vi "right2.vi"(10 "Parâmetros Ini 2":T2={"Gyro Port"=0, "Sensor - Left"=3, "Sensor - Right"=2, "     Color \nSensor Port"=1, "Kp Front"=0.5, "Motor speed"=-15, "Distance to street"=0.0, "Motor speed turns"=16, "Kp Curvas"=0.5} {"Kp Front" format="%.3f"; "Color \nSensor Port" items=["Port 1", "Port 2", "Port 3", "Port 4"]; "Sensor - Right" items=["Port 1", "Port 2", "Port 3", "Port 4"]; "Sensor - Left" items=["Port 1", "Port 2", "Port 3", "Port 4"]; "Gyro Port" items=["Port 1", "Port 2", "Port 3", "Port 4"]}, 11 "NXT/EV3":T1) -> (0 "x = y?":bool, 2 "NXT/EV3 2":T1)   [LabVIEW 2016]
uses:
  <vilib>/NXT/Subs/LVHSConnector.ctl
  <vilib>/NXT/LegoClasses/BrickReference/BrickReference.lvclass
  parametros.ctl
  <vilib>/NXT/Block Support/NXT_InputPort.ctl
  <vilib>/NXT/Block Support/NXT_OutputPort.ctl
  <vilib>/NXT/Dual Mode Library/Sensors/EV3_Gyro_Angle.vi
  <vilib>/NXT/NXTIO Xnodes/NXTIONodeSubVIs/NXTMoveMotors.vi
  <vilib>/NXT/NXTIO Xnodes/AddressXNode/NXTIOAddress.xnode
  <vilib>/NXT/NXTIO Xnodes/NXTIOXNode/NXTIO.xnode
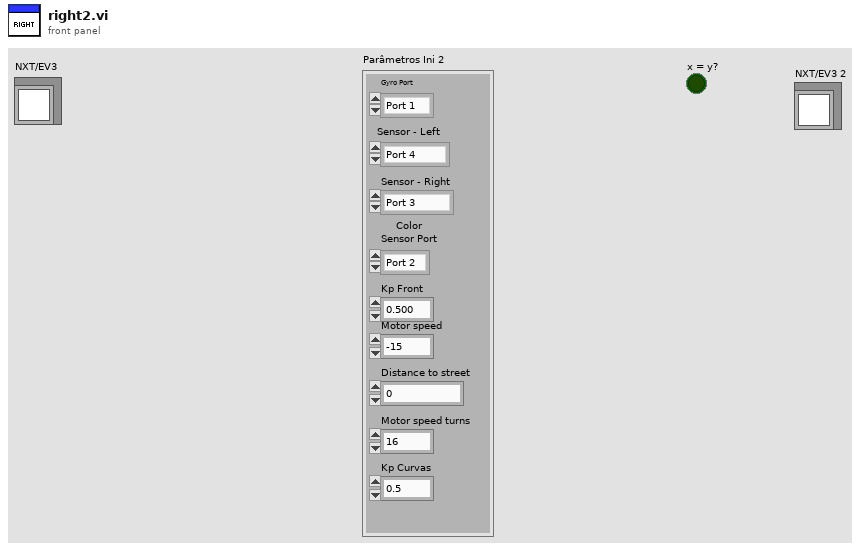
[diagram p1: front panel]
types:
  T1 = typedef "LVHSConnector.ctl" = refnum<class "BrickReference.lvclass">
  T2 = typedef "parametros.ctl" = cluster{"Gyro Port":T3, "Sensor - Left":T3, "Sensor - Right":T3, "     Color \nSensor Port":T3, "Kp Front":dbl, "Motor speed":i32, "Distance to street":dbl, "Motor speed turns":i32, "Kp Curvas":dbl}
  T3 = typedef "NXT_InputPort.ctl" = u32
  T4 = typedef "NXT_OutputPort.ctl" = u8
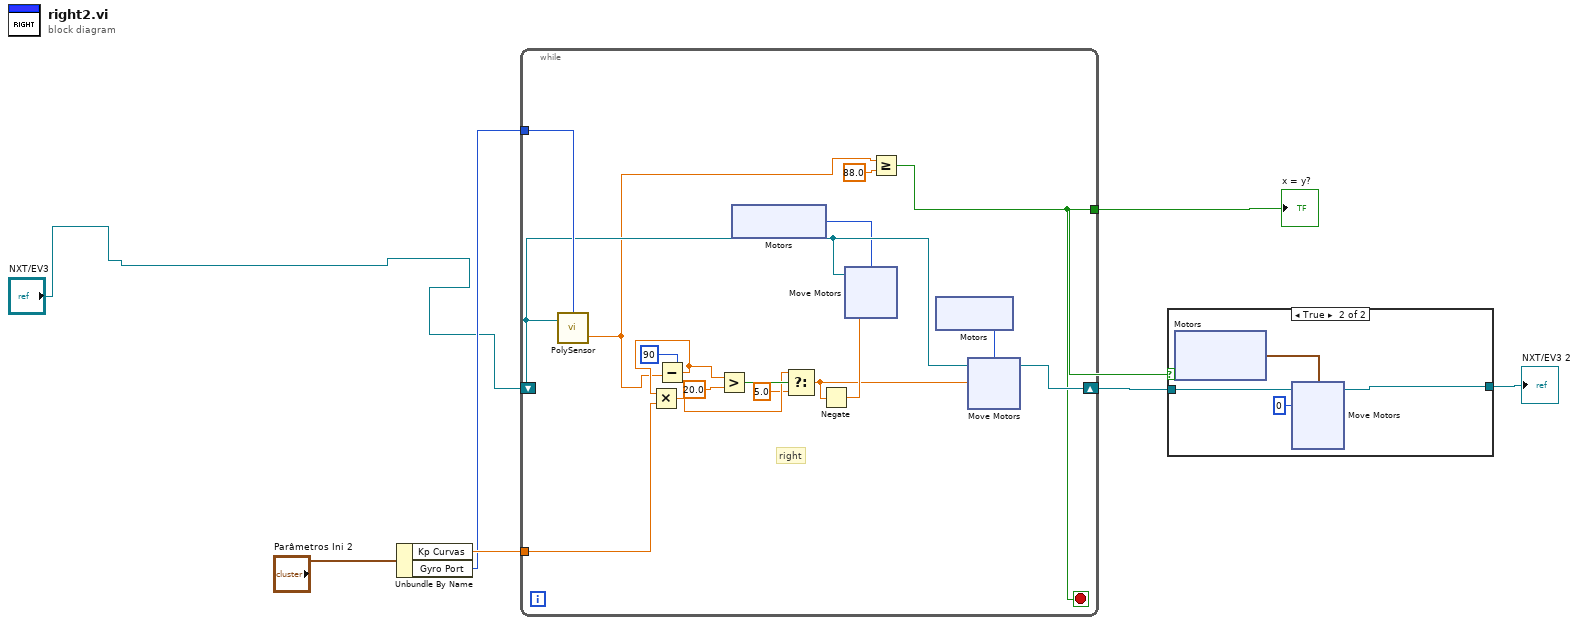
[diagram p0: block diagram]
diagram:
  n1 = Unbundle By Name("Parâmetros Ini 2") -> ("Kp Curvas"=w6:dbl, "Gyro Port"=w4:T3)
  n2 = while {
    tunnel: w6 -> [w24]
    tunnel: w4 -> [w23]
    tunnel: [w8] -> w1
    shift-right: [w9] -> w2
    shift-left: "NXT/EV3" -> [w22]
    stop <- w8 stop-if-true
    # "right"
    n3 = call-poly <vilib>:"PolySensor.vi"("NXT/EV3"=w22, "Port (Port 1)"=w23) -> ("Degrees"=w12:sgl)  [unwired: 1 in, 1 out]
    n4 = Subtract(x=90, y=w12) -> (x-y=w15:sgl)
    n5 = Multiply(x=w15, y=w24) -> (x*y=w14:dbl)
    n6 = Greater?(x=w15, y=sgl 20.0) -> (0:w19:bool)
    n7 = xnode "Motors"() -> ("Motor"=w17:T4)
    n8 = Select(t=w14, s=w19, f=5.0) -> (s? t:f=w10:dbl)
    n9 = Negate(x=w10) -> (-x=w11:dbl)
    n10 = xnode "Move Motors"("Power/Speed 1"=w11, "Motors"=w17, "NXT/EV3"=w22) -> ()  [unwired: 1 out]
    n11 = Greater Or Equal?(x=w12, y=sgl 88.0) -> (x >= y?=w8:bool)
    n12 = xnode "Motors"() -> ("Motor"=w16:T4)
    n13 = xnode "Move Motors"("Power/Speed 1"=w10, "Motors"=w16, "NXT/EV3"=w22) -> ("NXT/EV3"=w9:T1)
  }
  "x = y?" <- w1
  n14 = case shown="True" w1 {
    tunnel: w2 -> [w41 w44]
    tunnel: [w41 w43] -> w5
    frame False {
    }
    frame True {
      w42 = i8 0 ("Power/Speed 1")
      n15 = xnode "Motors"() -> ("Motor"=w45:cluster{"Port":T4, "Port":T4})
      n16 = xnode "Move Motors"("Power/Speed 2"=w42, "Power/Speed 1"=w42, "Motors"=w45, "NXT/EV3"=w44) -> ("NXT/EV3"=w43:T1)
    }
  }
  "NXT/EV3 2" <- w5
